vi "Add-Ex-Mod-Manualy.vi"(6 "In_Sp_Init_Amnt":string[](array[string]), 8 "In-Ex_Mod_IDs":string[](array[string])=["LacI", "TetR"], 9 "In-Idx of Mod in Sp IDs":i32[](array[numeric]), 10 "Rest_Sp_IDs":string[](array[string]), 11 "Sp IDs":string[](array[string])) -> (0 "Out-Rest_Sp_Init_Amnt":string[](array[string]), 1 "Out-Ex_Mod_IDs":string[](array[string])=["LacI", "TetR"], 2 "O/p Idx of Mod in Sp IDs":i32[](array[numeric])=[1, 4], 3 "Out_Rest_Sp_IDs":string[](array[string]))   [LabVIEW 2014]
doc: "This VI is used to select the name of species which a user wants to make the external controls of. \n\nDesigned by:\nHB\nhaba@dtu.dk"
panel:
  in  "Done":bool
  in  "Make external controls of:":i32(listbox)
  in  "Available species:":i32(listbox)
  # "Select species for external controls"
  # "Drag the name of species from left-hand box and drop it to right-hand box."
  # "-->"
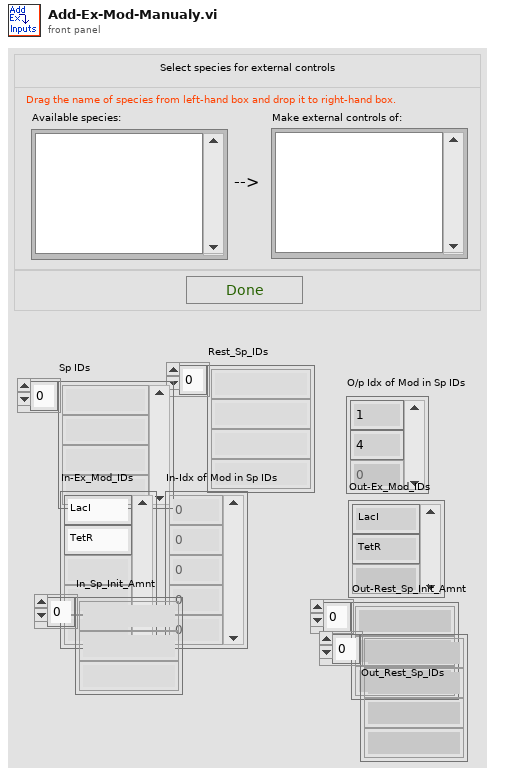
[diagram p1: front panel]
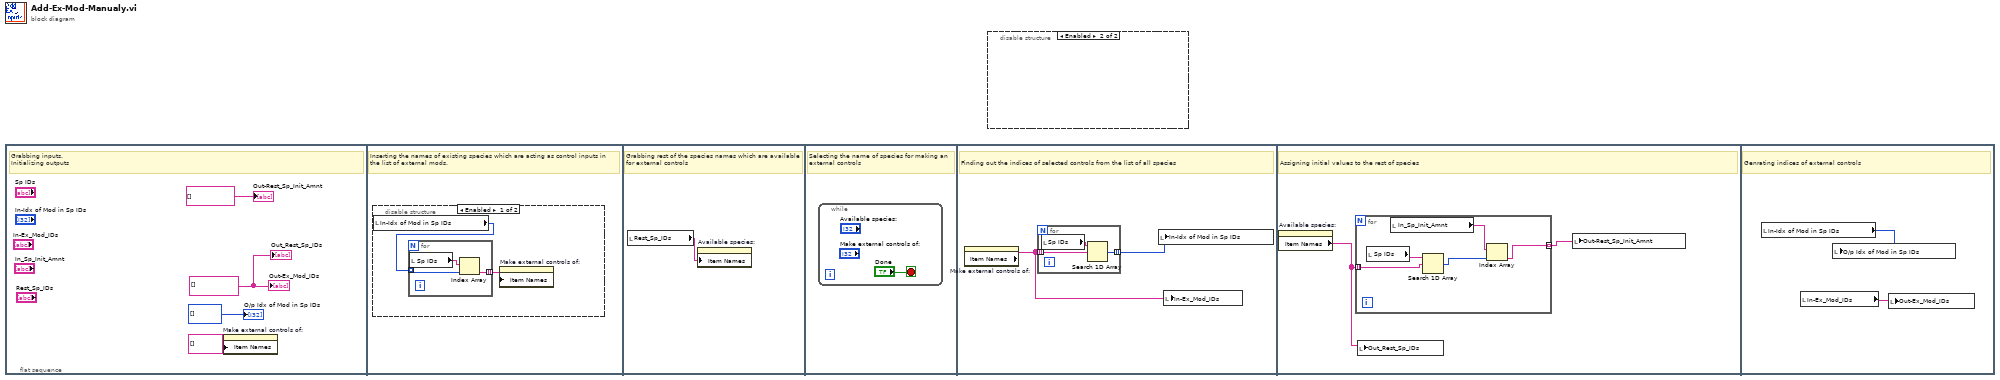
[diagram p0: block diagram]
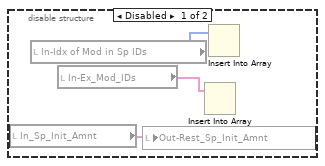
[diagram p2: hidden frame]
diagram:
  n1 = flat-sequence {
    frame #0 {
      w1 = string[] [] ("Ex_Mod_IDs")
      # "Grabbing inputs. \nInitializing outputs"
      n2 = property on="Make external controls of:" class="LstBox (strict)"("Item Names"=string[] []) -> ()  [unwired: 2 in, 2 out]
      "O/p Idx of Mod in Sp IDs" <- i32[] [] ("O/p Idx of Mod in Sp IDs")
      "Out-Ex_Mod_IDs" <- w1
      "Out-Rest_Sp_Init_Amnt" <- string[] [] ("Ex_Mod_IDs")
      "Out_Rest_Sp_IDs" <- w1
    }
    frame #1 {
      # "Inserting the names of existing species which are acting as control inputs in the list of external mods."
      n3 = disable-structure shown="Enabled" {
        frame Enabled {
          n4 = local read "In-Idx of Mod in Sp IDs"() -> (w6:i32[])
          n5 = for {
            tunnel: w6 -> [w8] mode=indexing
            tunnel: [w7] -> w5 mode=indexing
            n6 = local read "Sp IDs"() -> (w9:string[])
            n7 = Index Array(array=w9, index=w8) -> (element=w7:string)
          }
          n8 = property on="Make external controls of:" class="LstBox (strict)"("Item Names"=w5) -> ()  [unwired: 2 in, 2 out]
        }
        frame Disabled {
        }
      }
    }
    frame #2 {
      # "Grabbing rest of the species names which are available for external controls"
      n9 = local read "Rest_Sp_IDs"() -> (w10:string[])
      n10 = property on="Available species:" class="LstBox (strict)"("Item Names"=w10) -> ()  [unwired: 2 in, 2 out]
    }
    frame #3 {
      # "Selecting the name of species for making an external controls"
      n11 = while {
        stop <- "Done" stop-if-true
      }
    }
    frame #4 {
      # "Finding out the indices of selected controls from the list of all species"
      n12 = property on="Make external controls of:" class="LstBox (strict)"() -> ("Item Names"=w12:string[])  [unwired: 2 in, 2 out]
      n13 = for {
        tunnel: w12 -> [w16] mode=indexing
        tunnel: [w15] -> w13 mode=indexing
        n14 = local read "Sp IDs"() -> (w14:string[])
        n15 = Search 1D Array(1D array=w14, element=w16) -> (index of element=w15:i32)  [unwired: 1 in]
      }
      n16 = local write "In-Idx of Mod in Sp IDs"(w13) -> ()
      n17 = local write "In-Ex_Mod_IDs"(w12) -> ()
    }
    frame #5 {
      # "Assigning initial values to the rest of species"
      n18 = property on="Available species:" class="LstBox (strict)"() -> ("Item Names"=w17:string[])  [unwired: 2 in, 2 out]
      n19 = for {
        tunnel: w17 -> [w22] mode=indexing
        tunnel: [w19] -> w18 mode=indexing
        n20 = local read "Sp IDs"() -> (w23:string[])
        n21 = local read "In_Sp_Init_Amnt"() -> (w21:string[])
        n22 = Search 1D Array(1D array=w23, element=w22) -> (index of element=w20:i32)  [unwired: 1 in]
        n23 = Index Array(array=w21, index=w20) -> (element=w19:string)
      }
      n24 = local write "Out_Rest_Sp_IDs"(w17) -> ()
      n25 = local write "Out-Rest_Sp_Init_Amnt"(w18) -> ()
    }
    frame #6 {
      # "Genrating indices of external controls"
      n26 = local read "In-Idx of Mod in Sp IDs"() -> (w25:i32[])
      n27 = local read "In-Ex_Mod_IDs"() -> (w24:string[])
      n28 = local write "O/p Idx of Mod in Sp IDs"(w25) -> ()
      n29 = local write "Out-Ex_Mod_IDs"(w24) -> ()
    }
  }
  n30 = disable-structure shown="Enabled" {
    frame Disabled {
      n31 = local read "In_Sp_Init_Amnt"() -> (w26:string[])
      n32 = local read "In-Idx of Mod in Sp IDs"() -> (w28:i32[])
      n33 = local read "In-Ex_Mod_IDs"() -> (w27:string[])
      n34 = local write "Out-Rest_Sp_Init_Amnt"(w26) -> ()
      n35 = Insert Into Array(array=w27) -> ()  [unwired: 2 in, 1 out]
      n36 = Insert Into Array(array=w28) -> ()  [unwired: 2 in, 1 out]
    }
    frame Enabled {
    }
  }
